vi "SetCurrentScreen.vi"(8 "error in (no error)":errorcluster, 11 "Bouncer in":refnum<class "Bouncer.lvclass">) -> (0 "error out":errorcluster, 3 "Bouncer out":refnum<class "Bouncer.lvclass">)   [LabVIEW 2019, in "RT_Game.lvlib" / "Bouncer.lvclass"]
uses:
  Bouncer.lvclass
  C:/Users/FreshBob/Dropbox/VIs/myRIO_GameConsole/RT/RT_Game/Game/Game.lvclass
  Bouncer.lvclass/Bouncer.ctl
  BounceTarget/BounceTarget.lvclass/BounceTarget.ctl
  BounceTarget/Write DoDraw.vi
  Game/Game.lvclass
  BounceTarget/BounceTarget.lvclass
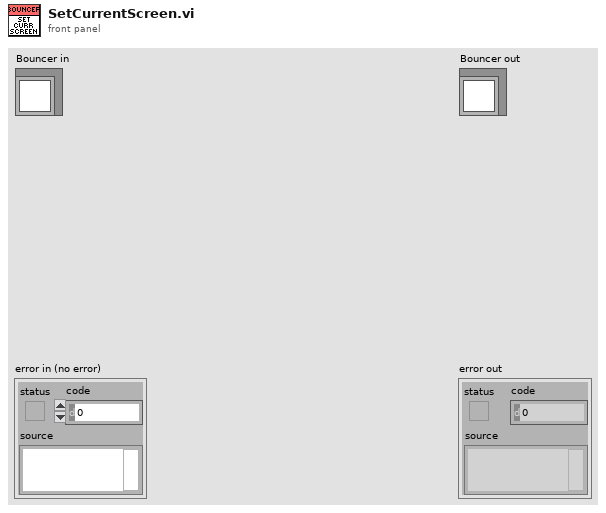
[diagram p1: front panel]
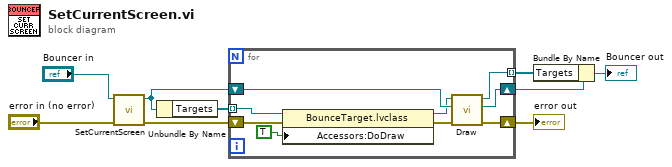
[diagram p0: block diagram]
diagram:
  n1 = call-parent "SetCurrentScreen.vi"("error in (no error)"="error in (no error)", "Game in"="Bouncer in") -> ("error out"=w4:errorcluster, "Game out"=w5:refnum<class "Bouncer.lvclass">)  [unwired: 8 in]
  n2 = Unbundle By Name(w5) -> ("Targets"=w6:refnum<class "BounceTarget.lvclass">[])
  n3 = for {
    tunnel: w6 -> [w12] mode=indexing
    shift-right: [w17] -> w2
    shift-left: w4 -> [w18]
    tunnel: [w16] -> w7 mode=indexing
    shift-right: [w15] -> w1
    shift-left: w5 -> [w14]
    n4 = property class="BounceTarget.lvclass"(reference=w12, error in=w18, "Accessors:DoDraw"=TRUE ("DoDraw")) -> (reference out=w11:refnum<class "BounceTarget.lvclass">, error out=w13:errorcluster)
    n5 = call "Draw.vi"("error in (no error)"=w13, "RT_Game.lvlib:Game.lvclass"=w14, "BounceTarget in"=w11) -> ("error out"=w17:errorcluster, "RT_Game.lvlib:Game.lvclass 2"=w15:refnum<class "Bouncer.lvclass">, "BounceTarget out"=w16:refnum<class "BounceTarget.lvclass">)  [unwired: 6 in]
  }
  "error out" <- w2
  n6 = Bundle By Name(cluster=w1, "Targets"=w7) -> (→"Bouncer out":refnum<class "Bouncer.lvclass">)
